vi "LIA 4IIR.vi"(6 "lock-in.iir config0 0":T2={"b0"=0.015777587890625, "b1"=-0.030517578125, "-a1"=1.9578399658203125, "-a2"=-0.9589080810546875}, 7 "lock-in.iir enable0 0":bool, 9 "input valid":bool, 10 "lock-in.iir decimation0 0":fxp<+,4,4> format="%#_3g", 11 "IQ_Data_In":T1) -> (1 "output valid":bool, 3 "IQ_Data_Out":T1)   [LabVIEW 2017]
uses:
  Cascaded-SOS/FPGA/Controls/IIR_Coeffs.ctl
  <instrlib>/_niInstr/DSP/v1/Shared/Public/IQ Data.ctl
  <instrlib>/_niInstr/DSP/v1/Shared/niInstr DSP v1 Shared.lvlib
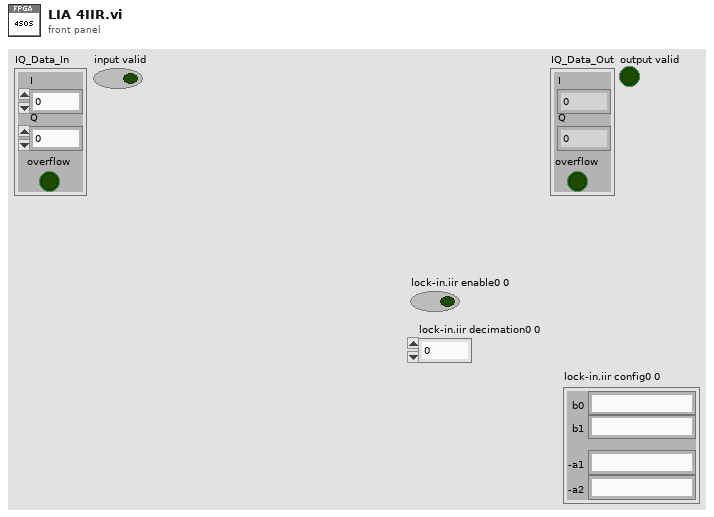
[diagram p1: front panel]
types:
  T1 = typedef "niInstr DSP v1 Shared.lvlib/IQ Data.ctl" = cluster{"I":fxp<+/-,18,1>, "Q":fxp<+/-,18,1>, "overflow":bool}
  T2 = typedef "IIR_Coeffs.ctl" = cluster{"b0":fxp<+/-,18,2>, "b1":fxp<+/-,18,2>, "-a1":fxp<+/-,18,2>, "-a2":fxp<+/-,18,2>}
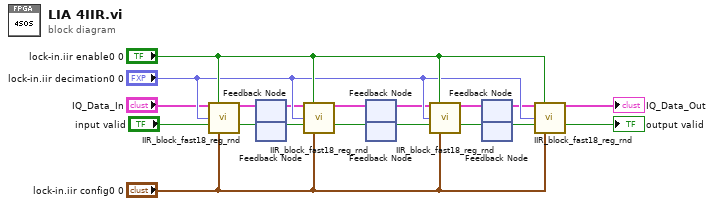
[diagram p0: block diagram]
diagram:
  n1 = call "IIR_block_fast18_reg_rnd.vi"("IQ_Data_In"="IQ_Data_In", "enable"="lock-in.iir enable0 0", "Decimation Factor (-1)"="lock-in.iir decimation0 0", "Valid In"="input valid", "IIR 2 coeffs"="lock-in.iir config0 0") -> ("IQ_Data_Out"=w19:T1, "output valid"=w16:bool)  [unwired: 9 in]
  n2 = feedback-in #1(w19) -> ()
  n3 = feedback #1() -> (w6:T1)  [unwired: 1 in]
  n4 = feedback-in #2(w16) -> ()
  n5 = feedback #2() -> (w5:bool)  [unwired: 1 in]
  n6 = call "IIR_block_fast18_reg_rnd.vi"("IQ_Data_In"=w6, "enable"="lock-in.iir enable0 0", "Decimation Factor (-1)"="lock-in.iir decimation0 0", "Valid In"=w5, "IIR 2 coeffs"="lock-in.iir config0 0") -> ("IQ_Data_Out"=w18:T1, "output valid"=w15:bool)  [unwired: 9 in]
  n7 = feedback-in #3(w18) -> ()
  n8 = feedback #3() -> (w4:T1)  [unwired: 1 in]
  n9 = feedback-in #4(w15) -> ()
  n10 = feedback #4() -> (w3:bool)  [unwired: 1 in]
  n11 = call "IIR_block_fast18_reg_rnd.vi"("IQ_Data_In"=w4, "enable"="lock-in.iir enable0 0", "Decimation Factor (-1)"="lock-in.iir decimation0 0", "Valid In"=w3, "IIR 2 coeffs"="lock-in.iir config0 0") -> ("IQ_Data_Out"=w17:T1, "output valid"=w14:bool)  [unwired: 9 in]
  n12 = feedback-in #5(w17) -> ()
  n13 = feedback #5() -> (w2:T1)  [unwired: 1 in]
  n14 = feedback-in #6(w14) -> ()
  n15 = feedback #6() -> (w1:bool)  [unwired: 1 in]
  n16 = call "IIR_block_fast18_reg_rnd.vi"("IQ_Data_In"=w2, "enable"="lock-in.iir enable0 0", "Decimation Factor (-1)"="lock-in.iir decimation0 0", "Valid In"=w1, "IIR 2 coeffs"="lock-in.iir config0 0") -> ("IQ_Data_Out"=→"IQ_Data_Out":T1, "output valid"=→"output valid":bool)  [unwired: 9 in]
